vi "Initialize Detector USB communication only has to run once after the ADconv is disconnected (SubVI).vi"(11 "VISA Refnum in":refnum<visa-resource-name>) -> (0 "error out":errorcluster, 1 "USB_Standard Configuration Descriptor":T1, 2 "USB_Standard Device Descriptor":T2 {"idProduct" format="%04x"; "idVendor" format="%04x"; "bcdUSB" format="%x"}, 3 "VISA Refnum out":refnum<visa-resource-name>)   [LabVIEW 2014]
uses:
  From internet/USB communication/Standard USB Functions/Standard Device Requests/Standard Descriptor Types/USB_Device Class.ctl
  From internet/USB communication/Standard USB Functions/Standard Device Requests/Standard Descriptor Types/USB_Standard Device Descriptor.ctl
  From internet/USB communication/Standard USB Functions/Standard Device Requests/Standard Descriptor Types/USB_Standard Configuration Descriptor.ctl
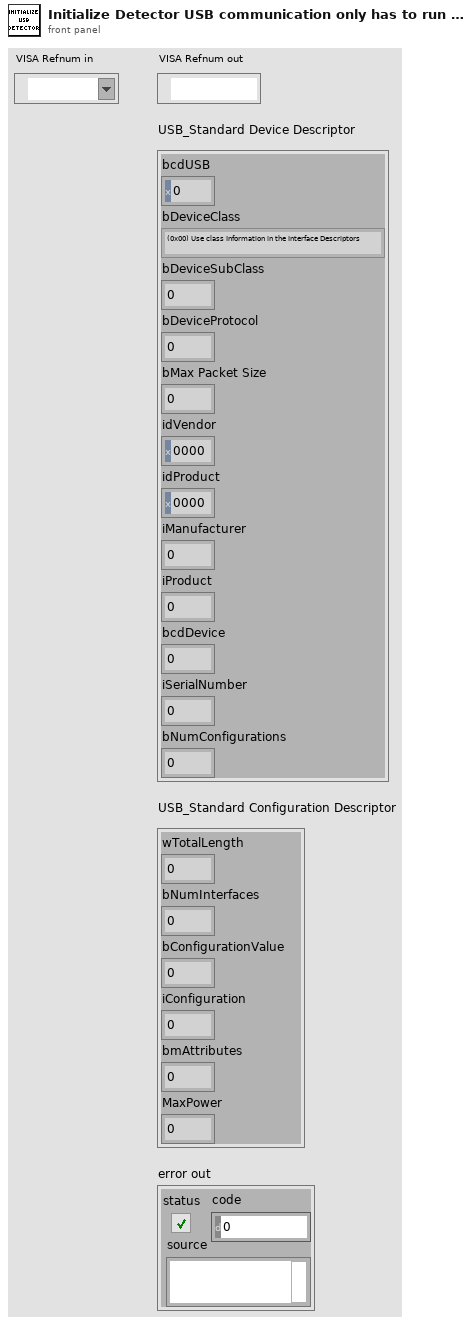
[diagram p1: front panel]
types:
  T1 = typedef "USB_Standard Configuration Descriptor.ctl" = cluster{"wTotalLength":u16, "bNumInterfaces":u8, "bConfigurationValue":u8, "iConfiguration":u8, "bmAttributes":u8, "MaxPower":u8}
  T2 = typedef "USB_Standard Device Descriptor.ctl" = cluster{"bcdUSB":u16, "bDeviceClass":T3, "bDeviceSubClass":u8, "bDeviceProtocol":u8, "bMax Packet Size":u8, "idVendor":u16, "idProduct":u16, "iManufacturer":u8, "iProduct":u8, "bcdDevice":u16, "iSerialNumber":u8, "bNumConfigurations":u8}
  T3 = typedef "USB_Device Class.ctl" = enum8{"(0x00) Use class Information in the Interface Descriptors", "(0x01) Audio", "(0x02) Communications and CDC Control", "(0x03) HID (Human Interface Device)", "(0x04) Reserved", "(0x05) Physical", "(0x06) Image", "(0x07) Printer", "(0x08) Mass Storage", "(0x09) Hub", "(0x0A) CDC-Data", "(0x0B) Smart Card", "(0x0C) Reserved", "(0x0D) Content Security", "(0x0E) Video", "(0x0F) Personal Healthcare", "(0x10) Reserved", "(0x11) Reserved", "(0x12) Reserved", "(0x13) Reserved", "(0x14) Reserved", "(0x15) Reserved", "(0x16) Reserved", "(0x17) Reserved", "(0x18) Reserved", "(0x19) Reserved", "(0x1A) Reserved", "(0x1B) Reserved", "(0x1C) Reserved", "(0x1D) Reserved", "(0x1E) Reserved", "(0x1F) Reserved", "(0x20) Reserved", "(0x21) Reserved", "(0x22) Reserved", "(0x23) Reserved", "(0x24) Reserved", "(0x25) Reserved", "(0x26) Reserved", "(0x27) Reserved", "(0x28) Reserved", "(0x29) Reserved", "(0x2A) Reserved", "(0x2B) Reserved", "(0x2C) Reserved", "(0x2D) Reserved", "(0x2E) Reserved", "(0x2F) Reserved", "(0x30) Reserved", "(0x31) Reserved", "(0x32) Reserved", "(0x33) Reserved", "(0x34) Reserved", "(0x35) Reserved", "(0x36) Reserved", "(0x37) Reserved", "(0x38) Reserved", "(0x39) Reserved", "(0x3A) Reserved", "(0x3B) Reserved", "(0x3C) Reserved", "(0x3D) Reserved", "(0x3E) Reserved", "(0x3F) Reserved", "(0x40) Reserved", "(0x41) Reserved", "(0x42) Reserved", "(0x43) Reserved", "(0x44) Reserved", "(0x45) Reserved", "(0x46) Reserved", "(0x47) Reserved", "(0x48) Reserved", "(0x49) Reserved", "(0x4A) Reserved", "(0x4B) Reserved", "(0x4C) Reserved", "(0x4D) Reserved", "(0x4E) Reserved", "(0x4F) Reserved", "(0x50) Reserved", "(0x51) Reserved", "(0x52) Reserved", "(0x53) Reserved", "(0x54) Reserved", "(0x55) Reserved", "(0x56) Reserved", "(0x57) Reserved", "(0x58) Reserved", "(0x59) Reserved", "(0x5A) Reserved", "(0x5B) Reserved", "(0x5C) Reserved", "(0x5D) Reserved", "(0x5E) Reserved", "(0x5F) Reserved", "(0x60) Reserved", "(0x61) Reserved", "(0x62) Reserved", "(0x63) Reserved", "(0x64) Reserved", "(0x65) Reserved", "(0x66) Reserved", "(0x67) Reserved", "(0x68) Reserved", "(0x69) Reserved", "(0x6A) Reserved", "(0x6B) Reserved", "(0x6C) Reserved", "(0x6D) Reserved", "(0x6E) Reserved", "(0x6F) Reserved", "(0x70) Reserved", "(0x71) Reserved", "(0x72) Reserved", "(0x73) Reserved", "(0x74) Reserved", "(0x75) Reserved", "(0x76) Reserved", "(0x77) Reserved", "(0x78) Reserved", "(0x79) Reserved", "(0x7A) Reserved", "(0x7B) Reserved", "(0x7C) Reserved", "(0x7D) Reserved", "(0x7E) Reserved", "(0x7F) Reserved", "(0x80) Reserved", "(0x81) Reserved", "(0x82) Reserved", "(0x83) Reserved", "(0x84) Reserved", "(0x85) Reserved", "(0x86) Reserved", "(0x87) Reserved", "(0x88) Reserved", "(0x89) Reserved", "(0x8A) Reserved", "(0x8B) Reserved", "(0x8C) Reserved", "(0x8D) Reserved", "(0x8E) Reserved", "(0x8F) Reserved", "(0x90) Reserved", "(0x91) Reserved", "(0x92) Reserved", "(0x93) Reserved", "(0x94) Reserved", "(0x95) Reserved", "(0x96) Reserved", "(0x97) Reserved", "(0x98) Reserved", "(0x99) Reserved", "(0x9A) Reserved", "(0x9B) Reserved", "(0x9C) Reserved", "(0x9D) Reserved", "(0x9E) Reserved", "(0x9F) Reserved", "(0xA0) Reserved", "(0xA1) Reserved", "(0xA2) Reserved", "(0xA3) Reserved", "(0xA4) Reserved", "(0xA5) Reserved", "(0xA6) Reserved", "(0xA7) Reserved", "(0xA8) Reserved", "(0xA9) Reserved", "(0xAA) Reserved", "(0xAB) Reserved", "(0xAC) Reserved", "(0xAD) Reserved", "(0xAE) Reserved", "(0xAF) Reserved", "(0xB0) Reserved", "(0xB1) Reserved", "(0xB2) Reserved", "(0xB3) Reserved", "(0xB4) Reserved", "(0xB5) Reserved", "(0xB6) Reserved", "(0xB7) Reserved", "(0xB8) Reserved", "(0xB9) Reserved", "(0xBA) Reserved", "(0xBB) Reserved", "(0xBC) Reserved", "(0xBD) Reserved", "(0xBE) Reserved", "(0xBF) Reserved", "(0xC0) Reserved", "(0xC1) Reserved", "(0xC2) Reserved", "(0xC3) Reserved", "(0xC4) Reserved", "(0xC5) Reserved", "(0xC6) Reserved", "(0xC7) Reserved", "(0xC8) Reserved", "(0xC9) Reserved", "(0xCA) Reserved", "(0xCB) Reserved", "(0xCC) Reserved", "(0xCD) Reserved", "(0xCE) Reserved", "(0xCF) Reserved", "(0xD0) Reserved", "(0xD1) Reserved", "(0xD2) Reserved", "(0xD3) Reserved", "(0xD4) Reserved", "(0xD5) Reserved", "(0xD6) Reserved", "(0xD7) Reserved", "(0xD8) Reserved", "(0xD9) Reserved", "(0xDA) Reserved", "(0xDB) Reserved", "(0xDC) Reserved", "(0xDD) Reserved", "(0xDE) Reserved", "(0xDF) Reserved", "(0xE0) Reserved", "(0xE1) Reserved", "(0xE2) Reserved", "(0xE3) Reserved", "(0xE4) Reserved", "(0xE5) Reserved", "(0xE6) Reserved", "(0xE7) Reserved", "(0xE8) Reserved", "(0xE9) Reserved", "(0xEA) Reserved", "(0xEB) Reserved", "(0xEC) Reserved", "(0xED) Reserved", "(0xEE) Reserved", "(0xEF) Reserved", "(0xF0) Reserved", "(0xF1) Reserved", "(0xF2) Reserved", "(0xF3) Reserved", "(0xF4) Reserved", "(0xF5) Reserved", "(0xF6) Reserved", "(0xF7) Reserved", "(0xF8) Reserved", "(0xF9) Reserved", "(0xFA) Reserved", "(0xFB) Reserved", "(0xFC) Reserved", "(0xFD) Reserved", "(0xFE) Reserved", "(0xFF) Reserved"}
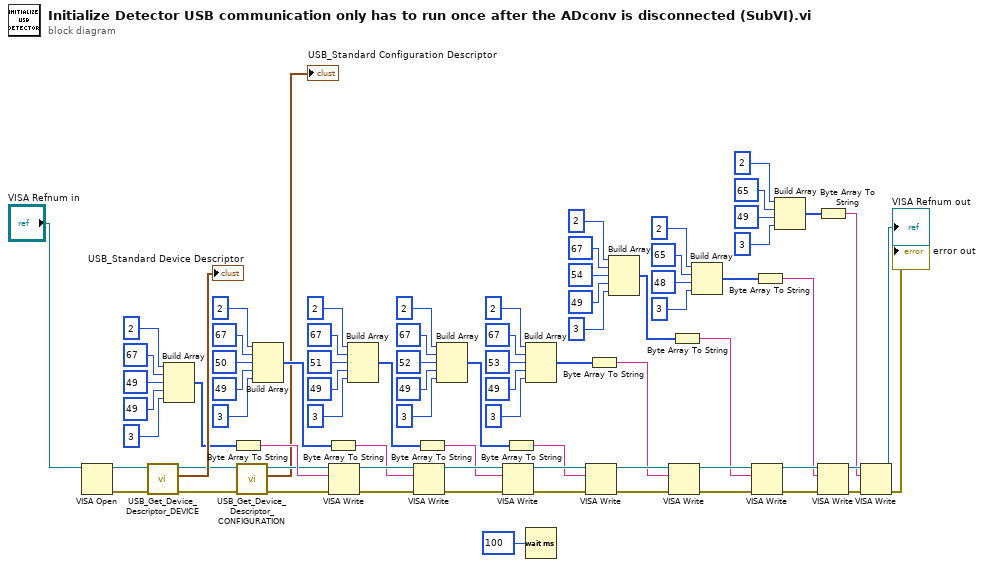
[diagram p0: block diagram]
diagram:
  n1 = VISA Open(VISA resource name="VISA Refnum in") -> (VISA resource name=w79:refnum<visa-resource-name>, error out=w78:errorcluster)  [unwired: 4 in]
  n2 = call "USB_Get_Device_Descriptor_DEVICE.vi"("error out 2"=w78, "VISA resource name"=w79) -> ("error out"=w5:errorcluster, "USB_bDescriptor Type 1"=→"USB_Standard Device Descriptor":T2, "VISA resource name 2"=w4:refnum<visa-resource-name>)  [unwired: 3 in]
  n3 = Build Array(2, 67, 49, 49, 3) -> (w58:i32[])
  n4 = Byte Array To String(unsigned byte array=w58) -> (string=w59:string)
  n5 = call "USB_Get_Device_Descriptor_CONFIGURATION.vi"("error out 2"=w5, "VISA resource name"=w4) -> ("error out"=w2:errorcluster, "USB_Standard Configuration Descriptor"=→"USB_Standard Configuration Descriptor":T1, "VISA resource name 2"=w3:refnum<visa-resource-name>)  [unwired: 2 in, 1 out]
  n6 = Build Array(2, 67, 50, 49, 3) -> (w51:i32[])
  n7 = Byte Array To String(unsigned byte array=w51) -> (string=w52:string)
  n8 = VISA Write(VISA resource name=w3, write buffer=w59, error in (no error)=w2) -> (VISA resource name out=w76:refnum<visa-resource-name>, error out=w75:errorcluster)  [unwired: 1 out]
  n9 = Build Array(2, 67, 51, 49, 3) -> (w44:i32[])
  n10 = VISA Write(VISA resource name=w76, write buffer=w52, error in (no error)=w75) -> (VISA resource name out=w74:refnum<visa-resource-name>, error out=w73:errorcluster)  [unwired: 1 out]
  n11 = Byte Array To String(unsigned byte array=w44) -> (string=w45:string)
  n12 = Build Array(2, 67, 52, 49, 3) -> (w37:i32[])
  n13 = VISA Write(VISA resource name=w74, write buffer=w45, error in (no error)=w73) -> (VISA resource name out=w72:refnum<visa-resource-name>, error out=w71:errorcluster)  [unwired: 1 out]
  n14 = Byte Array To String(unsigned byte array=w37) -> (string=w38:string)
  n15 = Build Array(2, 67, 53, 49, 3) -> (w30:i32[])
  n16 = Wait (ms)(milliseconds to wait=u32 100) -> ()  [unwired: 1 out]
  n17 = VISA Write(VISA resource name=w72, write buffer=w38, error in (no error)=w71) -> (VISA resource name out=w70:refnum<visa-resource-name>, error out=w69:errorcluster)  [unwired: 1 out]
  n18 = Byte Array To String(unsigned byte array=w30) -> (string=w31:string)
  n19 = Build Array(2, 67, 54, 49, 3) -> (w23:i32[])
  n20 = VISA Write(VISA resource name=w70, write buffer=w31, error in (no error)=w69) -> (VISA resource name out=w68:refnum<visa-resource-name>, error out=w67:errorcluster)  [unwired: 1 out]
  n21 = Byte Array To String(unsigned byte array=w23) -> (string=w24:string)
  n22 = Build Array(2, 65, 48, 3) -> (w16:i32[])
  n23 = VISA Write(VISA resource name=w68, write buffer=w24, error in (no error)=w67) -> (VISA resource name out=w66:refnum<visa-resource-name>, error out=w65:errorcluster)  [unwired: 1 out]
  n24 = Byte Array To String(unsigned byte array=w16) -> (string=w17:string)
  n25 = Build Array(2, 65, 49, 3) -> (w9:i32[])
  n26 = Byte Array To String(unsigned byte array=w9) -> (string=w10:string)
  n27 = VISA Write(VISA resource name=w66, write buffer=w17, error in (no error)=w65) -> (VISA resource name out=w64:refnum<visa-resource-name>, error out=w63:errorcluster)  [unwired: 1 out]
  n28 = VISA Write(VISA resource name=w64, write buffer=w10, error in (no error)=w63) -> (VISA resource name out=→"VISA Refnum out":refnum<visa-resource-name>, error out=→"error out":errorcluster)  [unwired: 1 out]
